vi "calc.vi"() -> ()   [LabVIEW 2022 SP3]
uses:
  SM_Data.ctl
  SM_States.ctl
panel:
  out "SM_Data":T1
  out "Display 2":dbl
  in  "Action Display":string
  in  "Actions":T2
  in  "Input":T3
  out "Display":dbl
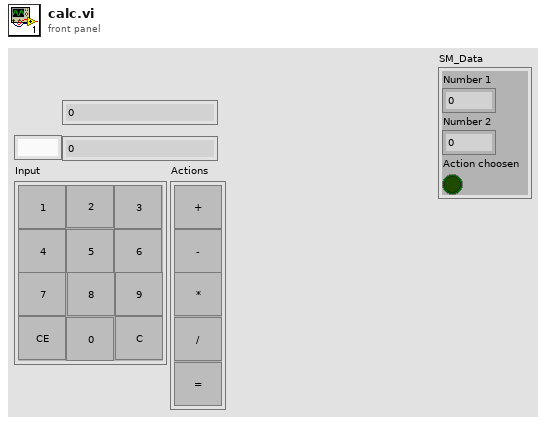
[diagram p1: front panel]
types:
  T1 = typedef "SM_Data.ctl" = cluster{"Number 1":dbl, "Number 2":dbl, "Action choosen":bool}
  T2 = cluster{"OK Button":bool, "OK Button 4":bool, "OK Button 7":bool, "OK Button 8":bool, "OK Button 9":bool}
  T3 = cluster{"OK Button":bool, "OK Button 2":bool, "OK Button 3":bool, "OK Button 4":bool, "OK Button 5":bool, "OK Button 6":bool, "OK Button 7":bool, "OK Button 8":bool, "OK Button 9":bool, "OK Button 10":bool, "OK Button 11":bool, "OK Button 12":bool}
  T4 = typedef "SM_States.ctl" = enum16{"Update Indicator", "Handle Action Press", "Handle Number Press", "Stop", "Initialize", "Idle"}
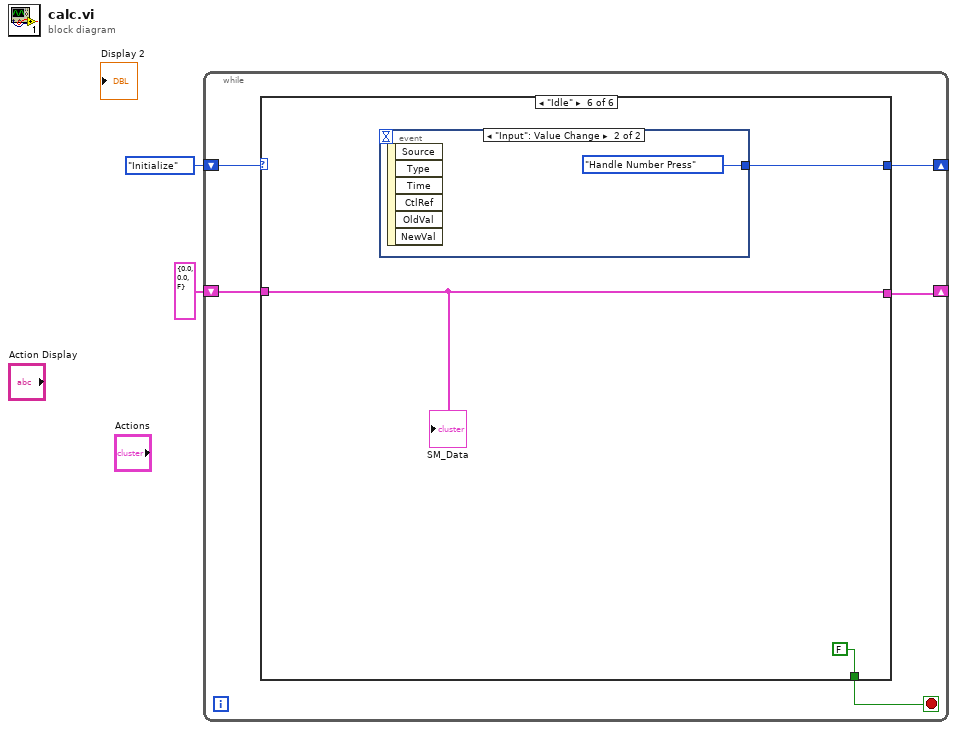
[diagram p0: block diagram]
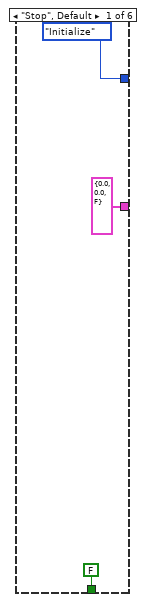
[diagram p2: hidden frame]
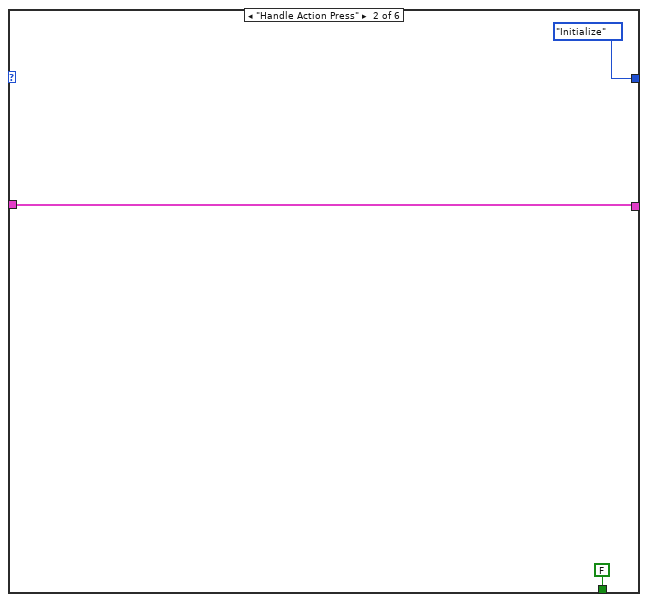
[diagram p3: hidden frame]
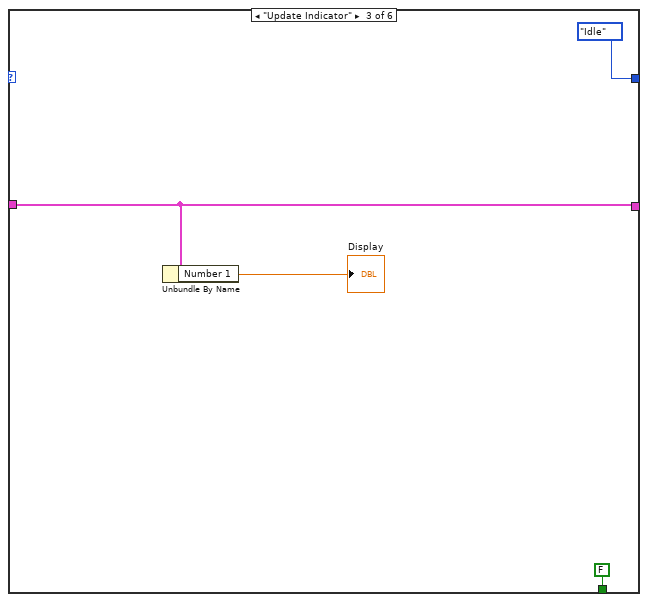
[diagram p4: hidden frame]
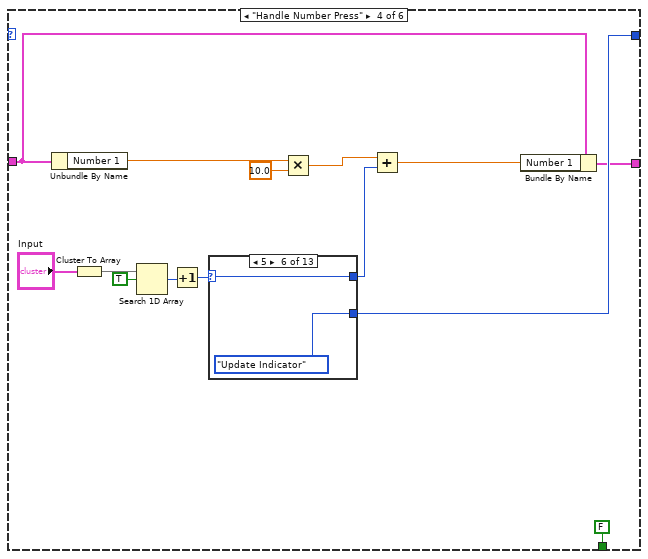
[diagram p5: hidden frame]
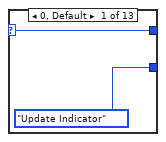
[diagram p6: hidden frame]
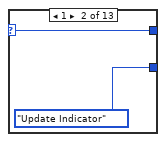
[diagram p7: hidden frame]
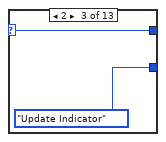
[diagram p8: hidden frame]
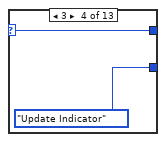
[diagram p9: hidden frame]
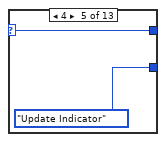
[diagram p10: hidden frame]
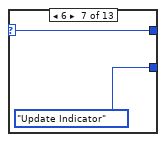
[diagram p11: hidden frame]
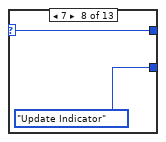
[diagram p12: hidden frame]
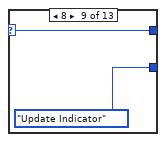
[diagram p13: hidden frame]
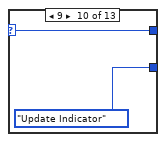
[diagram p14: hidden frame]
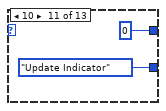
[diagram p15: hidden frame]
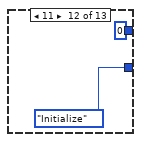
[diagram p16: hidden frame]
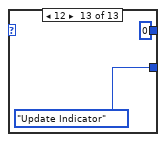
[diagram p17: hidden frame]
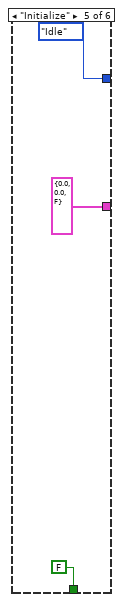
[diagram p18: hidden frame]
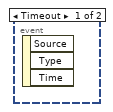
[diagram p19: hidden frame]
diagram:
  n1 = while {
    shift-right: [w6] -> _
    shift-left: SM_States."Initialize" ("SM_States") -> [w7]
    shift-right: [w5] -> _
    shift-left: T1 {"Number 1"=0.0, "Number 2"=0.0, "Action choosen"=FALSE} ("SM_Data") -> [w3]
    stop <- w4 stop-if-true
    n2 = case shown="\"Idle\"" w7 {
      tunnel: [SM_States."Initialize" ("SM_States") SM_States."Initialize" ("SM_States") SM_States."Idle" ("SM_States") w23 SM_States."Idle" ("SM_States") w63] -> w6
      tunnel: [T1 {"Number 1"=0.0, "Number 2"=0.0, "Action choosen"=FALSE} ("SM_Data") w11 w15 w21 T1 {"Number 1"=0.0, "Number 2"=0.0, "Action choosen"=FALSE} ("SM_Data") w61] -> w5
      tunnel: [FALSE FALSE FALSE FALSE FALSE FALSE] -> w4
      tunnel: w3 -> [_ w11 w15 w22 _ w61]
      frame "Stop", Default {
      }
      frame "Handle Action Press" {
      }
      frame "Update Indicator" {
        n3 = Unbundle By Name(w15) -> ("Number 1"=→"Display":dbl)
      }
      frame "Handle Number Press" {
        n4 = Unbundle By Name(w22) -> ("Number 1"=w20:dbl)
        n5 = Cluster To Array(cluster="Input") -> (array=w29:bool[])
        n6 = Search 1D Array(1D array=w29, element=TRUE) -> (index of element=w27:i32)  [unwired: 1 in]
        n7 = Increment(x=w27) -> (x+1=w26:i32)
        n8 = case shown="5" w26 {
          selector: w26 -> [w33 w35 w37 w39 w41 w43 w45 w47 w49 w51 _ _ _]
          tunnel: [w33 w35 w37 w39 w41 w43 w45 w47 w49 w51 0 ("index of element") 0 ("index of element") 0 ("index of element")] -> w18
          tunnel: [SM_States."Update Indicator" ("SM_States") SM_States."Update Indicator" ("SM_States") SM_States."Update Indicator" ("SM_States") SM_States."Update Indicator" ("SM_States") SM_States."Update Indicator" ("SM_States") SM_States."Update Indicator" ("SM_States") SM_States."Update Indicator" ("SM_States") SM_States."Update Indicator" ("SM_States") SM_States."Update Indicator" ("SM_States") SM_States."Update Indicator" ("SM_States") SM_States."Update Indicator" ("SM_States") SM_States."Initialize" ("SM_States") SM_States."Update Indicator" ("SM_States")] -> w23
          frame 0, Default {
          }
          frame 1 {
          }
          frame 2 {
          }
          frame 3 {
          }
          frame 4 {
          }
          frame 5 {
          }
          frame 6 {
          }
          frame 7 {
          }
          frame 8 {
          }
          frame 9 {
          }
          frame 10 {
          }
          frame 11 {
          }
          frame 12 {
          }
        }
        n9 = Multiply(x=w20, y=10.0) -> (x*y=w24:dbl)
        n10 = Add(x=w24, y=w18) -> (x+y=w19:dbl)
        n11 = Bundle By Name(cluster=w22, "Number 1"=w19) -> (w21:T1)
      }
      frame "Initialize" {
      }
      frame "Idle" {
        n12 = event shown="[1] \"Input\": Value Change" {
          selector: _ -> [_ _]
          dyn-events: _ -> [_ _]
          timeout: _ -> [_ _]
          tunnel: [_ SM_States."Handle Number Press" ("SM_States")] -> w63
          event Timeout {
            n13 = event-data() -> ()  [unwired: 1 in, 3 out]
          }
          event "Input": Value Change {
            n14 = event-data() -> ()  [unwired: 1 in, 6 out]
          }
        }
        "SM_Data" <- w61
      }
    }
  }
